vi "Get Thread Interface.vi"(10 "index":i32, 11 "Plugin in":refnum<class "Plugin.lvclass">) -> (2 "Plugin Interface":refnum<class "Plugin Interface.lvclass">, 3 "Plugin out":refnum<class "Plugin.lvclass">)   [LabVIEW 2019, in "DSF Core.lvlib" / "Plugin.lvclass"]
uses:
  Plugin.lvclass
  Interface/Plugin/Plugin Interface.lvclass
  Plugin.lvclass/Plugin.ctl
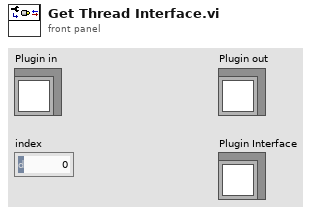
[diagram p1: front panel]
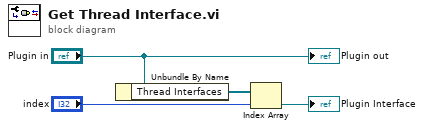
[diagram p0: block diagram]
diagram:
  n1 = Unbundle By Name("Plugin in") -> ("Thread Interfaces"=w3:refnum<class "Plugin Interface.lvclass">[])
  n2 = Index Array(array=w3, index="index") -> (element=→"Plugin Interface":refnum<class "Plugin Interface.lvclass">)
  "Plugin out" <- "Plugin in"
